vi "GOOP_UnInstallGDS.vi"(5 "error in (no error)":errorcluster) -> (19 "error out":errorcluster)   [LabVIEW 2020]
panel:
  out "_Progress":u8(slide) caption="Progress" scale=0.0..100.0
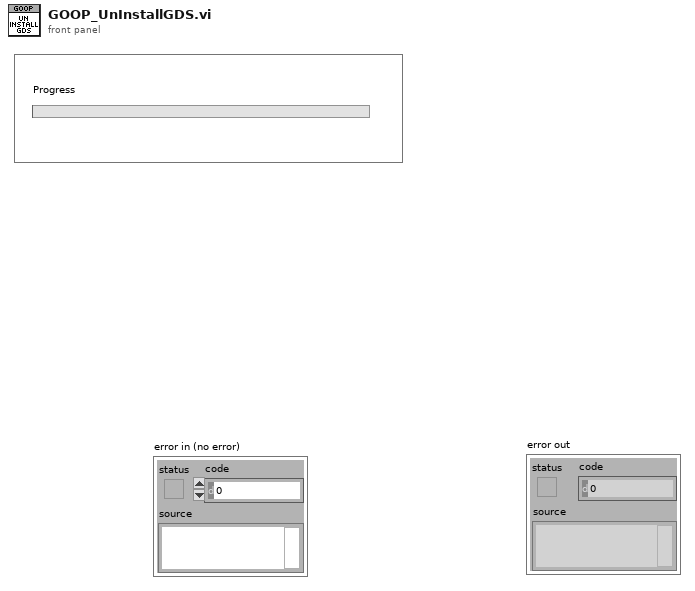
[diagram p1: front panel]
types:
  T1 = cluster{"All Folders":path[], "All Files in Dir":path[]}
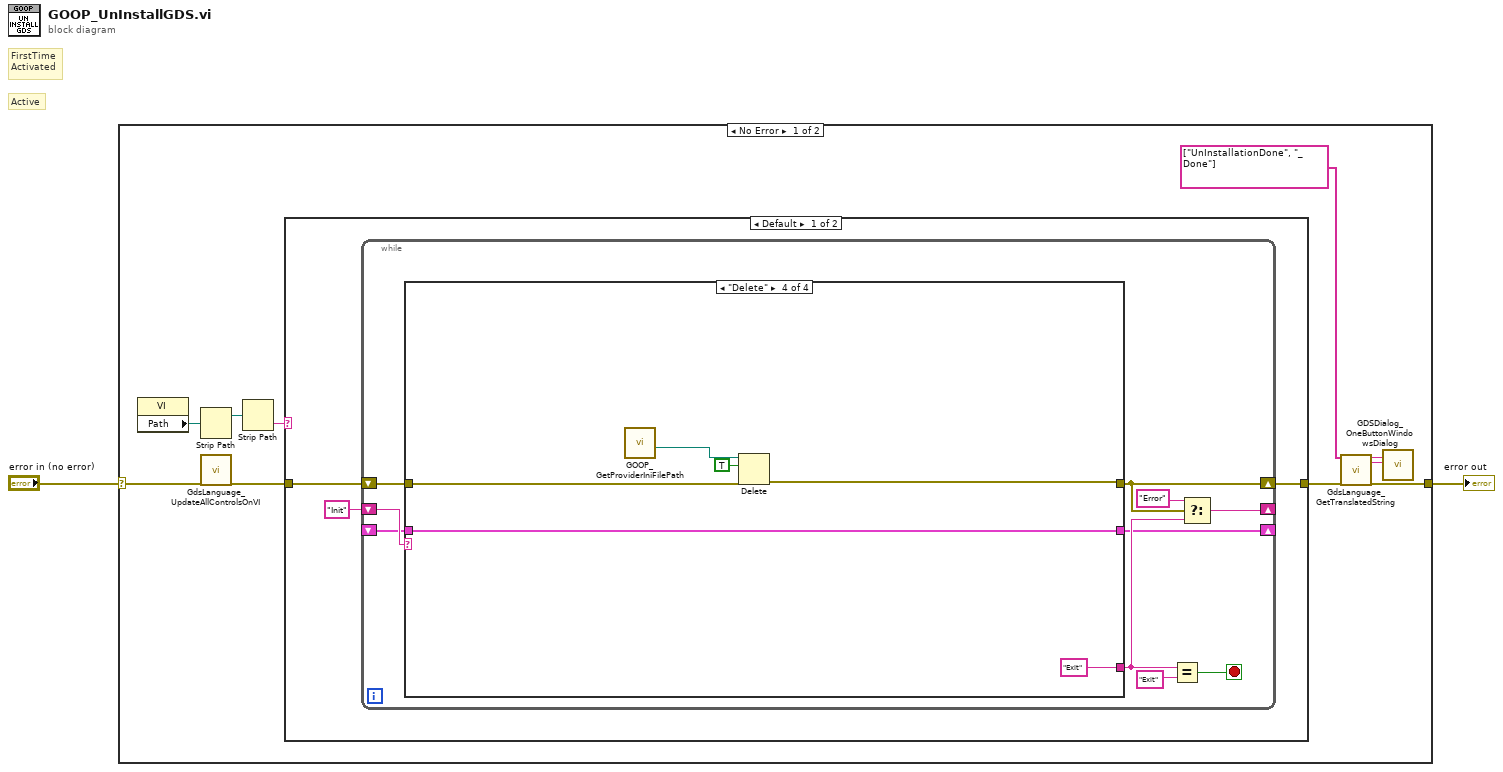
[diagram p0: block diagram]
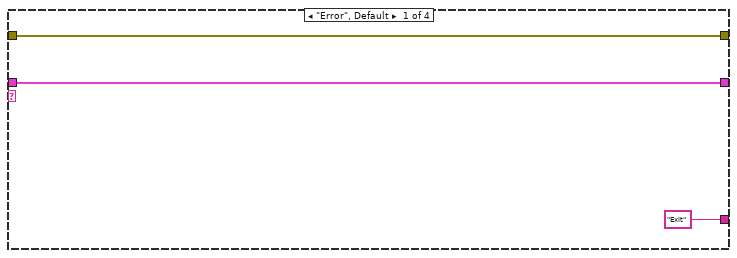
[diagram p2: hidden frame]
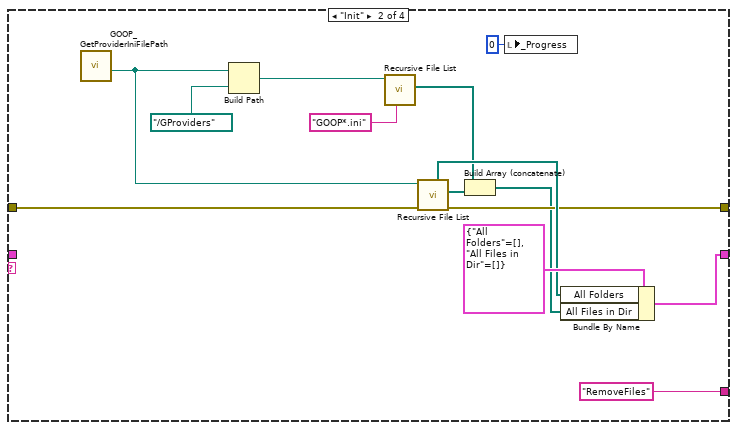
[diagram p3: hidden frame]
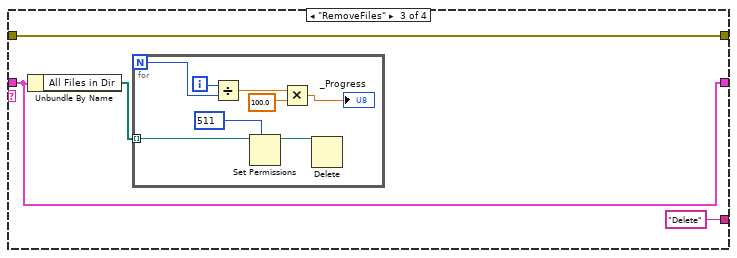
[diagram p4: hidden frame]
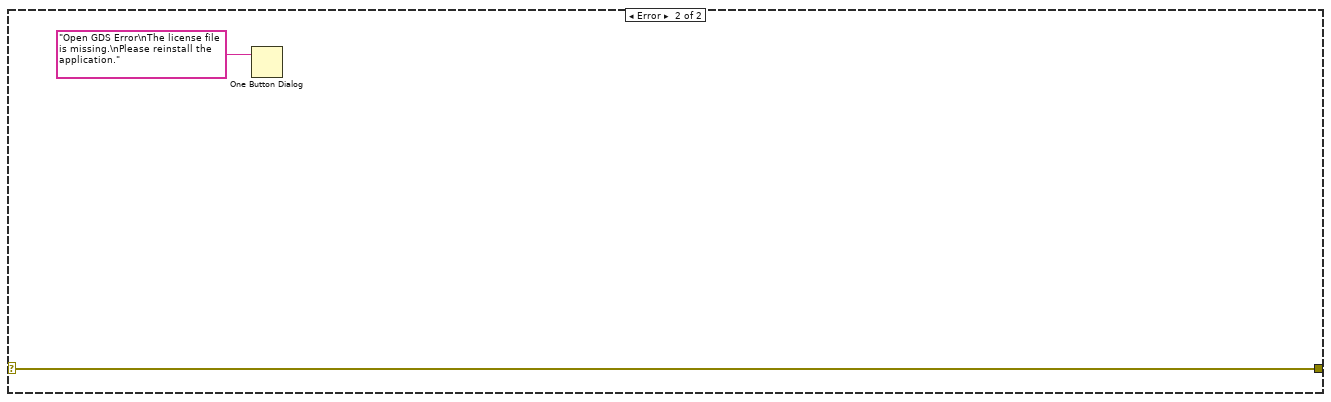
[diagram p6: hidden frame]
diagram:
  # "Active"
  # "FirstTime\nActivated"
  n1 = case shown="No Error" "error in (no error)" {
    selector: "error in (no error)" -> [w12 w62]
    tunnel: [w11 w62] -> w2
    frame No Error {
      n2 = property class="VI"() -> ("Path"=w5:path)  [unwired: 2 in, 2 out]
      n3 = Strip Path(path=w5) -> (stripped path=w6:path)  [unwired: 1 out]
      n4 = call "GdsLanguage_UpdateAllControlsOnVI.vi"("error in (no error)"=w12) -> ("error out"=w7:errorcluster)  [unwired: 17 in, 1 out]
      n5 = Strip Path(path=w6) -> (name=w4:string)  [unwired: 1 out]
      n6 = case shown="Default" w4 {
        tunnel: w7 -> [w14 w61]
        tunnel: [w13 w61] -> w3
        frame Default {
          n7 = while {
            shift-right: [w18] -> w13
            shift-left: w14 -> [w25]
            shift-right: [w23] -> _
            shift-left: "Init" -> [w24]
            shift-right: [w17] -> _
            shift-left: _ -> [w16]
            stop <- w22 stop-if-true
            n8 = case shown="\"Delete\"" w24 {
              tunnel: w25 -> [w28 w38 w44 w58]
              tunnel: [w28 w35 w44 w57] -> w18
              tunnel: ["Exit" "RemoveFiles" "Delete" "Exit"] -> w19
              tunnel: [w26 w40 w45 w59] -> w17
              tunnel: w16 -> [w26 _ w45 w59]
              frame "Error", Default {
              }
              frame "Init" {
                n9 = call "GOOP_GetProviderIniFilePath.vi"() -> ("ProviderMainFolder"=w29:path)  [unwired: 10 in, 1 out]
                n10 = Build Path(base path=w29, name or relative path=path "../GProviders" ("base path")) -> (appended path=w32:path)
                n11 = call <vilib>:"Recursive File List.vi"("pattern"="GOOP*.ini", "Folder Path"=w32) -> ("All Files in Dir"=w30:path[])  [unwired: 5 in, 4 out]
                n12 = call <vilib>:"Recursive File List.vi"("error in (no error)"=w38, "Folder Path"=w29) -> ("error out"=w35:errorcluster, "All Files in Dir"=w36:path[], "All Folders"=w37:path[])  [unwired: 5 in, 2 out]
                n13 = Build Array (concatenate)(w30, w36) -> (w31:path[])
                n14 = local write "_Progress"(u8 0 ("_Progress")) -> ()
                n15 = Bundle By Name(cluster=T1 {"All Folders"=[], "All Files in Dir"=[]}, "All Folders"=w37, "All Files in Dir"=w31) -> (w40:T1)
              }
              frame "RemoveFiles" {
                n16 = Unbundle By Name(w45) -> ("All Files in Dir"=w43:path[])
                n17 = for {
                  N -> [w53]
                  tunnel: w43 -> [w49] mode=indexing
                  i -> [w54]
                  n18 = Divide(x=w54, y=w53) -> (x/y=w52:dbl)
                  n19 = Set Permissions(7:i16 511 ("permissions"), 11:w49) -> (3:w47:path)  [unwired: 3 in, 1 out]
                  n20 = Multiply(x=w52, y=100.0) -> (x*y=→"_Progress":dbl)
                  n21 = Delete(path (use dialog)=w47) -> ()  [unwired: 4 in, 3 out]
                }
              }
              frame "Delete" {
                n22 = call "GOOP_GetProviderIniFilePath.vi"() -> ("ProviderMainFolder"=w56:path)  [unwired: 10 in, 1 out]
                n23 = Delete(path (use dialog)=w56, entire hierarchy (F)=TRUE, error in=w58) -> (error out=w57:errorcluster)  [unwired: 2 in, 2 out]
              }
            }
            n24 = Equal?(x=w19, y="Exit") -> (x = y?=w22:bool)
            n25 = Select(t="Error", s=w18, f=w19) -> (s? t:f=w23:string)
          }
        }
        frame "SubVIs" {
        }
      }
      n26 = call "GdsLanguage_GetTranslatedString.vi"("StringID(s)"=string[] ["UnInstallationDone", "_Done"], "error in (no error)"=w3) -> ("FirstStringOut"=w9:string, "SecondStringOut"=w8:string, "error out"=w11:errorcluster)  [unwired: 14 in, 1 out]
      n27 = call "GDSDialog_OneButtonWindowsDialog.vi"("UserText"=w9, "ButtonName"=w8) -> ()  [unwired: 15 in, 3 out]
    }
    frame Error {
      n28 = One Button Dialog(message="Open GDS Error\nThe license file is missing.\nPlease reinstall the application.") -> ()  [unwired: 1 in, 1 out]
    }
  }
  "error out" <- w2
